vi "Init.vi"(8 "error in (no error)":errorcluster, 11 "NI Vision Camera in":refnum<class "NI Vision Camera.lvclass">) -> (0 "error out":errorcluster, 3 "NI Vision Camera out":refnum<class "NI Vision Camera.lvclass">)   [LabVIEW 2014, in "NI Vision Camera.lvclass"]
uses:
  NI Vision Camera.lvclass
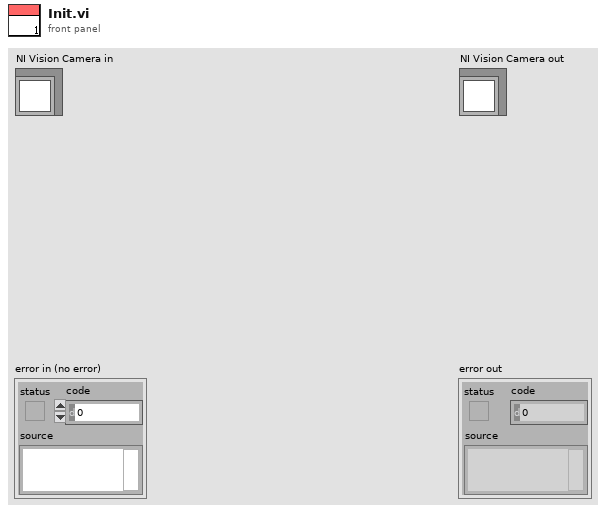
[diagram p1: front panel]
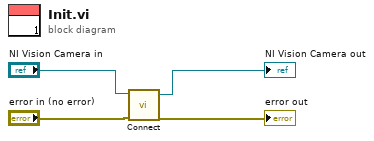
[diagram p0: block diagram]
diagram:
  n1 = call-dynamic "Connect.vi"("error in (no error)"="error in (no error)", "NI Vision Camera in"="NI Vision Camera in") -> ("error out"=→"error out":errorcluster, "NI Vision Camera out"=→"NI Vision Camera out":refnum<class "NI Vision Camera.lvclass">)  [unwired: 8 in]
